vi "Read Variables from the Dashboard.vi"() -> (3 "Dashboard Values":T1)   [LabVIEW 2017]
uses:
  <vilib>/Rock Robotics/Network Tables/NT Read Number.vi
  <vilib>/Rock Robotics/Network Tables/NT Read Boolean.vi
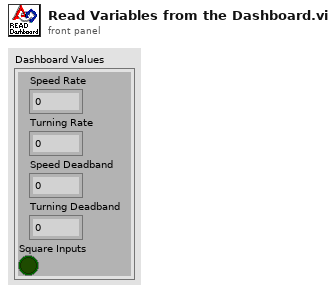
[diagram p1: front panel]
types:
  T1 = cluster{"Speed Rate":dbl, "Turning Rate":dbl, "Speed Deadband":dbl, "Turning Deadband":dbl, "Square Inputs":bool}
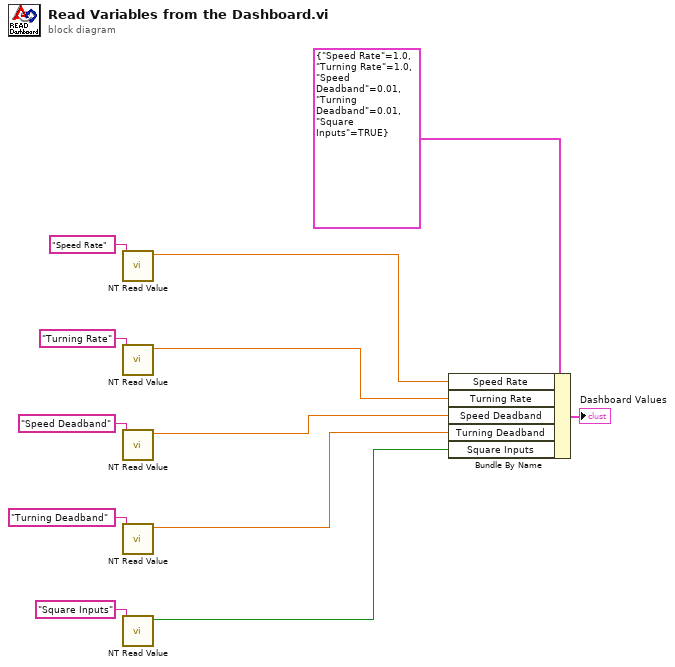
[diagram p0: block diagram]
diagram:
  n1 = call-poly <vilib>:"NT Read Value.vi"("Name"="Speed Rate") -> ("Numeric"=w6:dbl)  [unwired: 9 in, 1 out]
  n2 = call-poly <vilib>:"NT Read Value.vi"("Name"="Turning Rate") -> ("Numeric"=w5:dbl)  [unwired: 9 in, 1 out]
  n3 = call-poly <vilib>:"NT Read Value.vi"("Name"="Speed Deadband") -> ("Numeric"=w4:dbl)  [unwired: 9 in, 1 out]
  n4 = call-poly <vilib>:"NT Read Value.vi"("Name"="Turning Deadband") -> ("Numeric"=w3:dbl)  [unwired: 9 in, 1 out]
  n5 = call-poly <vilib>:"NT Read Value.vi"("Name"="Square Inputs") -> ("Boolean"=w2:bool)  [unwired: 9 in, 1 out]
  n6 = Bundle By Name(cluster=T1 {"Speed Rate"=1.0, "Turning Rate"=1.0, "Speed Deadband"=0.01, "Turning Deadband"=0.01, "Square Inputs"=TRUE}, "Speed Rate"=w6, "Turning Rate"=w5, "Speed Deadband"=w4, "Turning Deadband"=w3, "Square Inputs"=w2) -> (→"Dashboard Values":T1)
